vi "AlliGator Get Time Series Time Stamps & Settings from RecSettings Files.vi"(8 "Error In":errorcluster, 9 "Sorted Folder Names":string[](array[string]), 11 "Folder Path":path) -> (0 "Error Out":errorcluster, 1 "Time Stamps":dbl[](array[numeric]), 3 "Metadata String":string)   [LabVIEW 2021, in "AlliGator Files.lvlib"]
doc: "Extract time stamps of individual point in a series of LaVision FLI datasets."
uses:
  AlliGator Files.lvlib
panel:
  # "see the AlliGator License on the block diagram (Ctrl+E or Window:Show Block Diagram)"
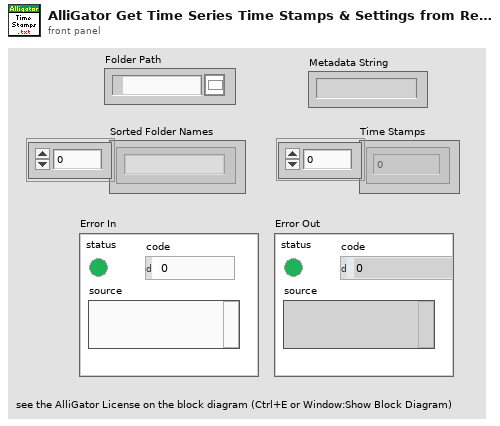
[diagram p1: front panel]
types:
  T1 = typedef "AlliGator Files.lvlib/AlliGator RecSettings Metadata.ctl" = cluster{"Time Stamp (s)":dbl, "First Gate":dbl[unit], "Gate Step":dbl[unit], "# Gates":i32, "Gate Duration":dbl[unit], "Laser Period":dbl[unit], "Gate Image Integration":dbl[unit], "Date":timestamp}
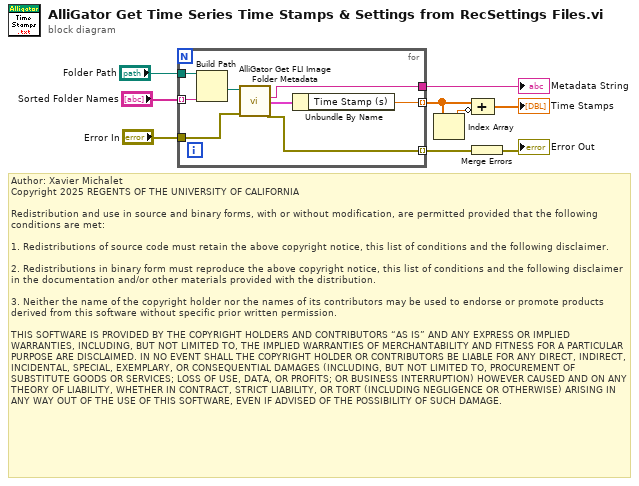
[diagram p0: block diagram]
diagram:
  # "Author: Xavier Michalet\nCopyright 2025 REGENTS OF THE UNIVERSITY OF CALIFORNIA\n\nRedistribution and use in source and binary forms, with or without modification, are permitted provided that the following conditions are met:\n\n1. Redistributions of source code must retain the above copyright notice, this list of conditions and the following disclaimer.\n\n2. Redistributions in binary form must reproduce the above copyright notice, this list of conditions and the following disclaimer in the documentation and/or other materials provided with the distribution.\n\n3. Neither the name of the copyright holder nor the names of its contributors may be used to endorse or promote products derived from this software without specific prior written permission.\n\nTHIS SOFTWARE IS PROVIDED BY THE COPYRIGHT HOLDERS AND CONTRIBUTORS “AS IS” AND ANY EXPRESS OR IMPLIED WARRANTIES, INCLUDING, BUT NOT LIMITED TO, THE IMPLIED WARRANTIES OF MERCHANTABILITY AND FITNESS FOR A PARTICULAR PURPOSE ARE DISCLAIMED. IN NO EVENT SHALL THE COPYRIGHT HOLDER OR CONTRIBUTORS BE LIABLE FOR ANY DIRECT, INDIRECT, INCIDENTAL, SPECIAL, EXEMPLARY, OR CONSEQUENTIAL DAMAGES (INCLUDING, BUT NOT LIMITED TO, PROCUREMENT OF SUBSTITUTE GOODS OR SERVICES; LOSS OF USE, DATA, OR PROFITS; OR BUSINESS INTERRUPTION) HOWEVER CAUSED AND ON ANY THEORY OF LIABILITY, WHETHER IN CONTRACT, STRICT LIABILITY, OR TORT (INCLUDING NEGLIGENCE OR OTHERWISE) ARISING IN ANY WAY OUT OF THE USE OF THIS SOFTWARE, EVEN IF ADVISED OF THE POSSIBILITY OF SUCH DAMAGE."
  n1 = for {
    tunnel: "Folder Path" -> [w17]
    tunnel: "Sorted Folder Names" -> [w16] mode=indexing
    tunnel: [w10] -> w7
    tunnel: [w15] -> w6 mode=indexing
    tunnel: "Error In" -> [w13]
    tunnel: [w12] -> w2 mode=indexing
    n2 = Build Path(base path=w17, name or relative path=w16) -> (appended path=w14:path)
    n3 = call "AlliGator Get FLI Image Folder Metadata.vi"("error in (no error)"=w13, "Image Folder in"=w14) -> ("error out"=w12:errorcluster, "Metadata"=w11:T1, "Metadata String"=w10:string)  [unwired: 6 in, 1 out]
    n4 = Unbundle By Name(w11) -> ("Time Stamp (s)"=w15:dbl)
  }
  "Metadata String" <- w7
  n5 = Index Array(array=w6) -> (element=w4:dbl)  [unwired: 1 in]
  n6 = Compound Arithmetic op=ADD(w6, invert w4) -> (→"Time Stamps":dbl[])
  n7 = Merge Errors(w2) -> (→"Error Out":errorcluster)
